vi "Test Glyph not Reset on Reload.vi"(8 "error in (no error)":errorcluster, 11 "Result Model Result Recording Test in":refnum<class "Result Model Result Recording Test.lvclass">) -> (0 "error out":errorcluster, 3 "Result Model Result Recording Test out":refnum<class "Result Model Result Recording Test.lvclass">)   [LabVIEW 2020, in "Result Model Result Recording Test.lvclass"]
uses:
  Result Model Result Recording Test.lvclass
  source/Core/Result/Type.ctl
  source/Core/Result/Result.lvlib
  source/Core/Result/Status.ctl
  source/Core/Result/Result.ctl
  source/User Interface/Result Model/Result Model.lvclass
  ae2c71b8-32bb-49d1-8500-0119bfec74ff.vi
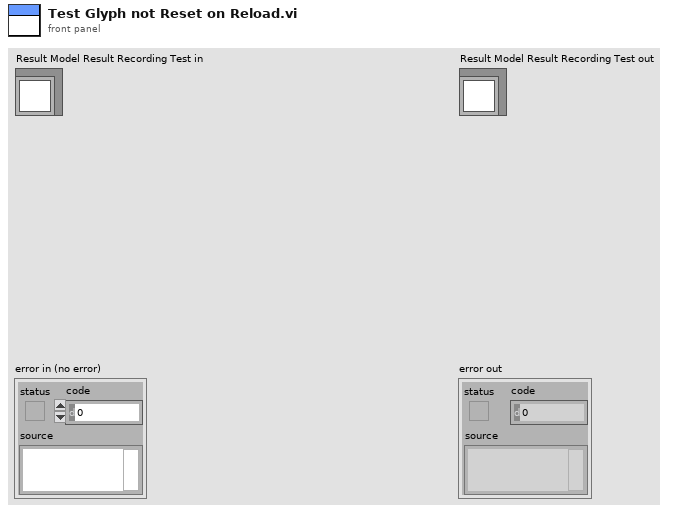
[diagram p1: front panel]
types:
  T1 = typedef "Result.lvlib/Result.ctl" = cluster{"Name":string, "Description":string, "Status":T2, "Result Type":T3, "Execution Time":dbl, "Data":cluster{"Expected":variant, "Actual":variant, "Delta":variant}}
  T2 = typedef "Result.lvlib/Status.ctl" = enum16{"", "Passed", "Failed", "Error", "Skipped", "Setup Error", "Broken", "Teardown Error"}
  T3 = typedef "Result.lvlib/Type.ctl" = enum16{"Test Case", "Test Suite", "Test Run", "Pass", "Fail", "Skip", "Pass if", "Fail if", "Pass if Error", "Fail if Error", "Pass if Equal", "Fail if Equal"}
  T4 = cluster{"Left Cell String":string, "Child Text":string[], "Child Tag":string, "Item Indent":i32, "Child Only?":bool, "Glyph Index":i32}[]
  T5 = cluster{"Left Cell String":string, "Child Text":string[], "Child Tag":string, "Item Indent":i32, "Child Only?":bool, "Glyph Index":i32}
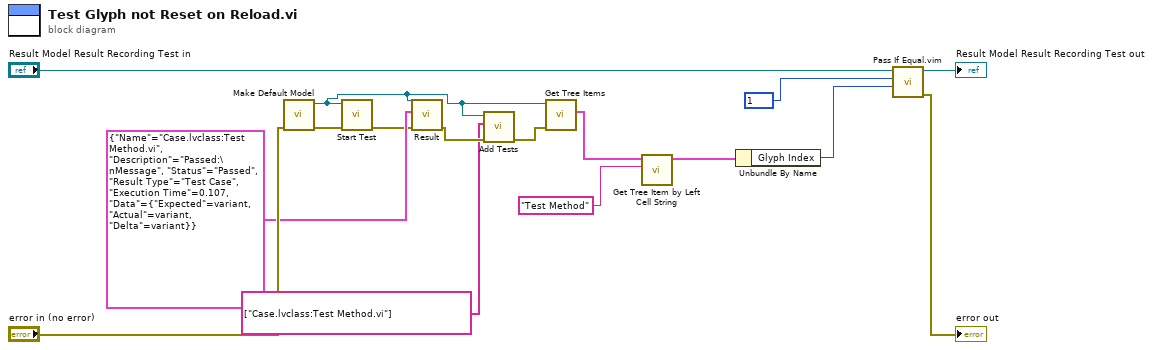
[diagram p0: block diagram]
diagram:
  n1 = call "Make Default Model.vi"("error in (no error)"="error in (no error)") -> ("error out"=w6:errorcluster, "Result Model out"=w4:refnum<class "Result Model.lvclass">)  [unwired: 9 in]
  n2 = call "Start Test.vi"("error in (no error)"=w6, "Result Model by Reference In"=w4) -> ("error out"=w5:errorcluster)  [unwired: 9 in]
  n3 = call-dynamic "Result.vi"("error in (no error)"=w5, "Results"=T1 {"Name"="Case.lvclass:Test Method.vi", "Description"="Passed:\nMessage", "Status"=enum."Passed", "Result Type"=enum."Test Case", "Execution Time"=0.107, "Data"={"Expected"=variant, "Actual"=variant, "Delta"=variant}} ("Result"), "Result Model by Reference In"=w4) -> ("error out"=w3:errorcluster)  [unwired: 8 in]
  n4 = call "Add Tests.vi"("error in (no error)"=w3, "Tests"=string[] ["Case.lvclass:Test Method.vi"], "Result Model by Reference In"=w4) -> ("error out"=w2:errorcluster)  [unwired: 8 in]
  n5 = call "Get Tree Items.vi"("error in (no error)"=w2, "Result Model by Reference In"=w4) -> ("Tree Items"=w16:T4)  [unwired: 8 in, 1 out]
  n6 = call "Get Tree Item by Left Cell String.vi"("Left Cell String"="Test Method", "Tree Items"=w16) -> ("Item"=w12:T5)  [unwired: 9 in]
  n7 = Unbundle By Name(w12) -> ("Glyph Index"=w11:i32)
  n8 = call "Pass If Equal.vim"("Actual"=w11, "Expected"=1 ("Listbox Symbol Ring Constant"), "LUnit Test Case In"="Result Model Result Recording Test in") -> ("error out"=→"error out":errorcluster, "LUnit Test Case Out"=→"Result Model Result Recording Test out":refnum<class "Result Model Result Recording Test.lvclass">)  [unwired: 7 in]
